vi "Example Monoflop.vi"() -> ()   [LabVIEW 2010]
uses:
  C:/tf/play/labview/Tinkerforge.dll
  Tinkerforge.dll
panel:
  in  "stop":bool
  in  "state":bool
  in  "uid":string="abc"
  in  "port":i32=4223
  in  "host":string="localhost"
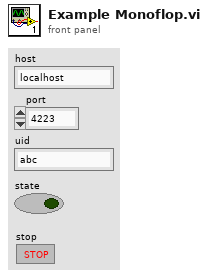
[diagram p1: front panel]
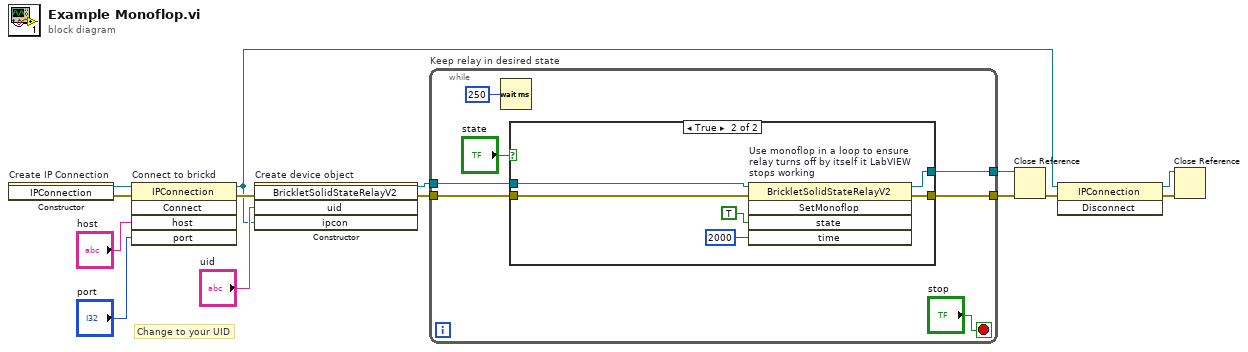
[diagram p0: block diagram]
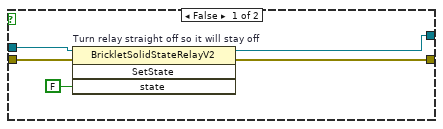
[diagram p2: hidden frame]
diagram:
  # "Change to your UID"
  n1 = constructor on="Create IP Connection" class="IPConnection"() -> (reference out=w14:refnum<k24>, error out=w5:errorcluster)  [unwired: 3 in, 1 out]
  n2 = invoke on="Connect to brickd" class="IPConnection" method="Connect"(reference=w14, error in=w5, "host"="host", "port"="port") -> (reference out=w7:refnum<k24>, error out=w10:errorcluster)  [unwired: 1 in, 3 out]
  n3 = constructor on="Create device object" class="BrickletSolidStateRelayV2"(error in=w10, "uid"="uid", "ipcon"=w7) -> (reference out=w3:refnum<k24>, error out=w4:errorcluster)  [unwired: 2 in, 3 out]
  n4 = while "Keep relay in desired state" {
    tunnel: w4 -> [w19]
    tunnel: [w18] -> w1
    tunnel: w3 -> [w17]
    tunnel: [w16] -> w2
    stop <- "stop" stop-if-true
    n5 = Wait (ms)(milliseconds to wait=u32 250) -> ()  [unwired: 1 out]
    n6 = case shown="True" "state" {
      tunnel: w19 -> [w25 w30]
      tunnel: [w24 w29] -> w18
      tunnel: w17 -> [w23 w28]
      tunnel: [w22 w27] -> w16
      frame False {
        n7 = invoke on="Turn relay straight off so it will stay off" class="BrickletSolidStateRelayV2" method="SetState"(reference=w23, error in=w25, "state"=FALSE) -> (reference out=w22:refnum<k24>, error out=w24:errorcluster)  [unwired: 1 in, 2 out]
      }
      frame True {
        n8 = invoke on="Use monoflop in a loop to ensure\nrelay turns off by itself it LabVIEW\nstops working" class="BrickletSolidStateRelayV2" method="SetMonoflop"(reference=w28, error in=w30, "state"=TRUE, "time"=i64 2000) -> (reference out=w27:refnum<k24>, error out=w29:errorcluster)  [unwired: 1 in, 3 out]
      }
    }
  }
  n9 = Close Reference(reference=w2, error in (no error)=w1) -> (error out=w9:errorcluster)
  n10 = invoke class="IPConnection" method="Disconnect"(reference=w7, error in=w9) -> (reference out=w6:refnum<k24>, error out=w8:errorcluster)  [unwired: 1 in, 1 out]
  n11 = Close Reference(reference=w6, error in (no error)=w8) -> ()  [unwired: 1 out]
